vi "LIA Example Host.vi"() -> ()   [LabVIEW 2017]
uses:
  Program Files (x86)/National Instruments/LabVIEW 2017/examples/Lock-In Amplifier/lib/host/Public/pll settings.ctl
  Program Files (x86)/National Instruments/LabVIEW 2017/examples/Lock-In Amplifier/lib/host/Public/lock-in settings.ctl
  Program Files (x86)/National Instruments/LabVIEW 2017/examples/Lock-In Amplifier/lib/interface/Interface FPGA/LIA Host Interface FPGA.lvclass
  C:/Program Files (x86)/National Instruments/LabVIEW 2017/examples/Lock-In Amplifier/lib/interface/Interface/LIA Host Interface.lvclass
  Program Files (x86)/National Instruments/LabVIEW 2017/examples/Lock-In Amplifier/lib/host/Public/fpga type.ctl
  Program Files (x86)/National Instruments/LabVIEW 2017/examples/Lock-In Amplifier/lib/interface/Interface FPGA/Properties/FpgaSession_GET.vi
  <vilib>/Utility/error.llb/Error Cluster From Error Code.vi
  <vilib>/rvi/errors/niLvFpgaAdjustHostInterfaceError.vi
  <vilib>/rvi/interface/nirviReadWriteControl/nirviReadWriteControl.xnode
  Program Files (x86)/National Instruments/LabVIEW 2017/examples/Lock-In Amplifier/lib/interface/Interface/LIA Host Interface.lvclass
  Program Files (x86)/National Instruments/LabVIEW 2017/examples/Lock-In Amplifier/lib/host/Lock-In Amplifier Example Host.lvlib
  Program Files (x86)/National Instruments/LabVIEW 2017/examples/Lock-In Amplifier/lib/shared/Lock-In Amplifier Example Shared.lvlib
  NiFpgaLv.dll
  <vilib>/rvi/interface/Simulation/niFpgaSimulationCallBeginRW.vi
panel:
  in  "trigger slope 1":enum16{"Positive", "Negative"}(ring)
  in  "lowLevel 1":dbl caption="pll.q 2" format="%#_6f"
  in  "highLevel 1":dbl=0.25 caption="pll.q 2" format="%#_6f"
  in  "trigger slope 0":enum16{"Positive", "Negative"}(ring)
  in  "lowLevel 0":dbl caption="pll.q 2" format="%#_6f"
  in  "highLevel 0":dbl=0.25 caption="pll.q 2" format="%#_6f"
  out "pll.vco output 0":fxp<+/-,49,1>=0.5 format="%0^#1_8g"
  out "pll.q 2":dbl=0.5 format="%#_6pV"
  out "Waveform Graph":cluster{"f0":dbl, "df":dbl, "magnitude":dbl[]}[](graph)=[{"f0"=0.0, "df"=48828.125, "magnitude"=[-46.93833321413425, -48.890085398745086, -57.05864793570993, -63.948010145782, -57.10808944274945, -63.55723661730865, -57.477633254873524, -63.388970771981256, -57.83858653215573, -63.04278294236552, -58.310732731480286, -62.75659424633111, -59.01913953160205, -62.55034509450798, -59.76806715246457, -62.45290461669743, -60.67593939903783, -62.55360847730091, -61.80337052022501, -62.7503089432639, -62.95874542404657, -63.17666796807587, -64.24815178765463, -63.58179265883102, -65.96263589732504, -64.29834519828907, -67.76706631207706, -65.25530419899528, -69.69720964445415, -66.48978075872667, -72.0836829037614, -67.87758710008302, -74.95546090477261, -70.02468767091023, -78.46318325872932, -72.61789596314395, -82.74302220692796, -76.45363219872509, -86.93156331597662, -81.93411626073177, -89.39593580415576, -99.6170681323641, -88.66324403386615, -83.63767905833946, -86.78510178329685, -77.97514394138707, -83.83057336078254, -74.91042135055551, -81.5475507560879, -73.50059696206921, -78.86254697144325, -72.13420582514291, -77.68352683311363, -71.47125092202423, -75.95623700109, -71.27989762649543, -74.95441595981052, -71.25879209888319, -73.9595113284693, -71.56173669996721, -73.54477863881124, -72.29773534656574, -73.22367389861854, -72.96381308648769, -72.9988078797969, -73.86835428297962, -72.95305526553327, -75.2471462028992, -73.52456103236882, -76.90120154185578, -74.35415308379046, -78.75438807181995, -75.52159448517878, -81.97850502570516, -77.0522962144752, -83.72534671678167, -79.22667312669566, -87.72245228429632, -82.41997364153613, -92.98958808340201, -88.94092629488937, -99.50542487601304, -104.43928510750062, -96.68595945743522, -89.84335052432984, -91.19624554856414, -83.82262417189582, -90.01723416008254, -80.15754604679948, -85.81708298956508, -78.30065773404802, -85.06593198935606, -77.23628138343811, -82.71304646807387, -76.35856258445034, -81.61855339489769, -75.96594028137565, -80.15275231432624, -75.79741810419392, -78.97129025392613, -75.86427195094097, -78.17458456209165, -76.12085849656066, -77.85383262432903, -76.74912507995519, -77.25671541218556, -77.8982284228998, -77.8212535613011, -78.99364420828655, -77.9535986594113, -80.5765883437286, -78.71247862445587, -82.81330063919576, -79.90075393045993, -84.51582581828501, -80.84734822816016, -88.15097620058117, -83.06948686637503, -90.43795841683013, -87.05804894598725, -100.9044462888944, -91.16184483511006, -99.25318703849094, -113.00302254650566, -101.23938945826266, -94.74360211928621, -93.60935601063579, -86.60563663892235, -90.06499901122993, -82.85388280403822, -89.22123700503676, -81.17742163079215, -87.46988992571065, -80.0064748842741, -85.67242615027025, -79.5534829705813, -85.2386741467478, -78.36875630953557, -83.74067249570277, -78.58966459550572, -82.65136916700945, -78.45793002426842, -81.60291278830285, -78.78545275144468, -81.44873599291637, -79.46689782726857, -80.9546312968039, -80.34286350947234, -80.64680657897753, -81.40467594015718, -81.45416553874705, -82.91913176326895, -82.01356243362385, -84.4698494074905, -82.43677736126503, -86.83038860613686, -84.19971850756579, -89.09446672366998, -85.50637044704303, -93.27140345100959, -90.41560771649186, -102.15908510562295, -94.5879404286508, -103.56313351942903, -113.25509523061405, -96.25338657002342, -93.35849714429017, -94.3068008800362, -88.27873675614035, -93.30083233782412, -85.39601004639363, -91.46280056925573, -83.25477812069862, -89.43703075785405, -82.62438364466891, -88.2225308674539, -81.04566563419816, -87.59003295267959, -80.9135761936175, -85.77827427186253, -80.22308425470746, -85.54716936739837, -80.30173677397998, -84.2175901500595, -80.56732874040298, -83.37768242883448, -81.48306367425042, -83.8906905917171, -82.20138677185858, -83.36581337182099, -83.25360739403229, -83.86719108117094, -85.13623924398044, -84.60141920705034, -85.63247211425215, -84.61891754501954, -89.11219644534478, -86.93675308563888, -90.65086474060264, -86.91978227755536, -94.32232024107083, -91.1937031528676, -105.67835131078319, -96.01996999749672, -108.19743564556381, -102.1759528334099, -98.13408028328126, -95.42561864673883, -103.03927558417618, -93.13041820570994, -92.61599840933886, -87.41561823576637, -95.6167947640217, -85.45482114157137, -89.26172625327284, -83.64736821155725, -90.73728201983252, -82.95136175993244, -90.47704364999184, -83.00757026802304, -89.1024095672369, -82.29357706840872, -88.23475300940171, -82.03587331514377, -86.85968342180617, -82.35711341553477, -85.81709753106743, -82.79370712523529, -85.95880792378041, -84.08514911178878, -86.24056528669705, -84.26663563351609, -85.11149144200135, -85.48335371583636, -85.92142581813184, -86.91808359752399, -86.58865058087574, -89.98286982647136, -87.49532734785518, -91.95474837719652, -89.34803145467214, -94.49767349488376, -92.45873563416424, -108.8690430269248, -98.69933253742657, -105.06246392868492, -111.38768449697511, -96.99118510161742, -95.28935999072544, -99.57447315645048, -91.921208747929, -94.58067683198153, -89.26115689307557, -95.97632975434266, -87.71112562159823, -95.6026253040889, -86.8643653685995, -94.03413185014664, -84.75458821373303, -90.53152615195356, -84.18265238198386, -90.74003839355723, -83.81237200473785, -88.98630392767043, -83.46732671915824, -88.80833466935512, -84.3729693934194, -89.09540947774846, -84.11269221746572, -87.01477738659764, -85.46574647387061, -88.82633557926184, -85.30529533094341, -86.64432037411572, -88.38882956922036, -89.46178094867575, -88.65167305541695, -89.05173580146197, -90.56355933624823, -89.78350226994066, -93.12832102157176, -91.52067729309718, -99.30869554872353, -94.87507585179671, -103.34143765953752, -100.85184172648087, -122.81434116496578, -106.73815887001018, -100.4378952074342, -102.02001564406744, -97.52306851355098, -94.56940172267517, -96.76524495433301, -89.94805427338399, -97.3848170465787, -88.86035744990033, -94.19234755063327, -86.61835716903454, -91.20282103849767, -85.07595457318845, -91.55874293944323, -85.03788023396316, -91.60457024090475, -84.46215997256039, -90.57121250734171, -84.83435358765959, -90.33972168032196, -84.4873262300197, -89.24140029984238, -85.1352382372926, -88.70896083363503, -85.5975672934432, -89.12875853347873, -86.53505382308096, -89.60175411890748, -88.0071551620068, -89.28181547323886, -89.27126299467224, -89.37796771473032, -91.7125863209184, -91.52209806412742, -93.2645811544421, -91.18984143652762, -95.81363430158875, -93.62301569519619, -104.16775936541315, -104.90602312527591, -113.16700957432688, -116.28917731958283, -101.96572273705183, -98.41482687439297, -99.72098919139918, -94.22144853044513, -95.01564070694563, -94.17707694153272, -94.02287362186925, -89.58355059750363, -98.92261465033643, -89.02859420719695, -94.68073466314038, -86.44103147442705, -91.90373963098203, -86.4749062880022, -94.84153506645869, -86.32943545083764, -91.60215019601517, -86.2323824481995, -92.02155272951049, -85.9972623610034, -91.32387548251664, -85.588514296591, -91.53470648146998, -86.2096134918317, -90.35669055111491, -88.00287392840076, -90.12141751973901, -89.44766457872662, -91.62087976611487, -91.05208067549513, -92.06362797535392, -91.10989004012806, -92.02930632263177, -97.8326419437665, -100.36369914302273, -96.71323750153027, -96.77554535749293, -104.0483458530803, -100.02615902224633, -107.35748572388934, -107.18491846666, -111.2107942940795, -101.34493721885849, -96.18458817889217, -95.05818354852602, -97.34815447051216, -92.36349598065061, -95.78385348959006, -89.7086230203063, -93.2365210743273, -88.04737944359495, -95.39968104514571, -88.1751912031278, -94.33963358398256, -86.96835690829943, -94.3448391909962, -87.94543163312412, -92.90493597746648, -87.22030009538193, -92.61262896853015, -86.30586131244313, -91.96103440057696, -86.7710521640438, -92.10322890271088, -88.8099510544229, -93.31727026496762, -88.39915058817098, -92.9724660735097, -89.53892755878542, -93.5679390287161, -92.14368535308965, -93.89854406383924, -93.06540499762073, -95.3716098006777, -96.36846381712701, -93.63623239819597, -99.39911564797553, -98.40395825782761, -100.94269872968796, -100.48369232950719, -104.96898067375994, -114.335263021867, -101.40187975001979, -98.65627818089435, -106.58072970493392, -104.44376560744413, -95.83027356701794, -92.97753215916143, -101.26434292825368, -93.50367975283709, -93.37263244117777, -89.44861935863923, -95.343734550422, -89.99933130658839, -99.99527004643943, -88.94925644025324, -93.18301244517464, -88.50885338097075, -95.18084024984185, -87.20676030200416, -95.23926810467589, -87.09957224800853, -92.1757639701081, -88.10417272814877, -94.72106133839601, -87.7772108681502, -92.91109610741583, -89.72414668122461, -93.22742894203847, -91.63186037346222, -95.68890880122552, -90.18179583705027, -93.59223328781121, -92.50281370390375, -94.04741609159348, -95.5573835037378, -97.19098591462304, -99.76079766259453, -98.20546781981285, -120.67183723001071, -103.20327161610481, -117.22027024101293, -105.09645279442447, -111.76755429121258, -113.04120386427974, -100.65061200309104, -96.88654432109547, -94.60215846035042, -93.49825828753863, -97.1667542174504, -94.38236741729683, -96.783281591943, -92.939285616442, -95.42524341021134, -89.7310231461323, -96.61418552254929, -89.15181635406329, -93.97977001970317, -89.25630669378194, -99.16812248160959, -89.40549989469969, -97.02103373489075, -88.08117642000238, -96.17212999699518, -87.76166390724612, -93.64057438170258, -88.20421502757773, -94.63414445257587, -89.48275213078753, -92.03704873153879, -91.18822814375747, -94.02753580779823, -92.25046023804195, -94.18472031424919, -95.7912337432503, -97.17361952054567, -97.57189526176677, -96.93431865585318, -102.04551967744064, -98.01984334480733, -97.80936648544454, -96.58319851428925, -103.08073994551233, -110.00167882027728, -108.52196994994446, -105.04853402419212, -101.33233085003278, -100.05040433917165, -99.22073393358865, -97.90929268980324, -98.89113225851989, -94.89288879112064, -97.93384172752636, -93.22419277669928, -96.01960899562502, -90.96253017735826, -94.32065948649546, -90.18255956439114, -94.9243761616897, -88.73145096365911, -95.65826240076106, -90.10091760259287, -98.3156872459785, -88.97172432282879, -94.68357816611993, -89.22286435681411, -96.33113850492892, -90.27256468692858, -97.52356475116345, -92.28994918400562, -96.39548763580854, -90.89270553951194, -95.24683746449244, -92.28348737753878, -94.54135448918169, -92.42301671907596, -96.24508547590521, -99.44340135136264, -100.90085793594595, -101.8210082553093, -100.62139348876947, -107.75005082456524, -101.18792193308998, -100.62321402005587, -106.14445292006377, -105.83949578053429, -107.80632506741767, -102.54660223569036, -108.59151037419879, -96.90782677416453, -100.64769899514724, -98.90076837905437, -96.2725953153946, -100.63869480989204, -93.57497128631536, -97.48996544980523, -92.0598771078806, -97.43531529596639, -91.70896750245781, -97.62553199959177, -89.90453042801695, -98.1895558530371, -91.28563260418011, -96.58606769664732, -89.6602652167721, -97.63127451658008, -90.06188532337133, -96.88320254636814, -92.10434711550748, -102.83415328605342, -91.97522523546786, -96.69674529333655, -91.54555505247494, -96.45677376279522, -94.40105972915326, -99.06442453405175, -95.85784268220618, -100.11209838032768, -96.3666970525114, -100.25033668665256, -101.63701920876531, -101.33176509769909, -108.49220907293285, -105.20698869391131, -108.51201611499555, -110.56213658974848, -103.88286882354619, -107.29652775251672, -100.21199149373265, -102.84474849090422, -105.38837926677445, -101.63659463064025, -100.19927788160382, -95.8841790949619, -99.06159894948496, -93.83003777289345, -98.62241277299339, -93.41972484372512, -96.85163908187218, -92.22305012467251, -98.30931966050954, -91.01393465151821, -96.6610842279197, -93.01366348474153, -99.40254068724771, -91.98688250178945, -97.8197024210045, -90.34022028730962, -95.26212499971268, -90.48623787418245, -97.28501156955554, -93.02707841894987, -99.4242294058617, -93.78403579509337, -102.4058010943352, -92.81743718612427, -97.25554725609649, -97.04610938164143, -104.56111849036819, -101.9867276361093, -103.69614871490393, -104.74168040294428, -100.60066394657342, -102.48071416087461, -104.83064451058839, -107.26658041556234, -110.00503214084297, -103.90297408190925, -109.56149727793942, -103.52026679181287, -103.90051784161805, -102.01215965881818, -103.34803834159351, -98.0276145235799, -96.38035775134539, -97.3546077254475, -94.31453760099365, -99.30006326184404, -96.25250684947787, -96.12470450005495, -91.57830601960927, -94.56483812993685, -91.7611403679199, -100.05865004766831, -92.84402279338929, -95.8657101518119, -91.81837191684286, -96.8413097745885, -89.99396126510099, -100.6611154167793, -93.47882774662997, -101.6552886734432, -91.90487651880966, -97.29970250454008, -95.48622404677303, -100.41640918017757, -94.80515000968441, -98.5276945872201, -100.73609481029864, -98.04340547902302, -96.88540783402982, -103.44300868430581, -99.6601137575993, -104.35594220885358, -109.94922945338091, -109.10632479160674, -107.76641232941655, -105.2450226453189, -99.91265402083279, -99.95270124336952, -101.3299547913052, -99.96894232524801, -100.36365349460627, -102.86784602376038, -98.02737777122191, -96.17199616892495, -96.8931790371181, -95.96337763969792, -97.57196266275315, -95.0155693239098, -97.04855005360989, -94.47249259707691, -99.4517730137364, -92.94791202171595, -97.78312777875891, -94.30168526906485, -94.86398262799752, -93.54115309153002, -99.87583067187317, -92.51726891229963, -102.13604597983688, -92.17994531242135, -101.63856277413217, -95.35318079876619, -99.29709984960036, -95.35866979801156, -103.51166947626271, -94.86370220831154, -101.60407867882681, -103.74156718150365, -110.73370380070999, -103.71760139847281, -107.37490721838113, -109.9542240510403, -116.25403765775846, -108.23241740959084, -105.09846687198814, -105.44052253244195, -115.24118791748435, -103.49001515992114, -110.71286352533042, -105.89441442611357, -110.16493279526881, -99.82773652058825, -98.97179081977004, -98.45757481371732, -98.24962705928117, -96.73193799282699, -96.5175230963137, -96.15492740611579, -95.37412981355675, -103.58492432555138, -95.34117451236305, -97.11997617370957, -93.47520800696678, -110.25299719363927, -96.81885358127444, -99.9145312135518, -94.20482495341496, -98.89579295580432, -93.36303704542247, -100.68935843408086, -93.24714444319031, -100.69789100599222, -95.91175346020901, -104.76997205430096, -94.51143912041329, -100.54159089868858, -102.05805669840157, -99.78073889500477, -95.8994839656266, -104.44581361115654, -97.35459561709312, -102.43458217795424, -99.94756951585332, -116.63154202021275, -104.67083143207799, -105.9908001506922, -110.38171109041919, -112.65697869449573, -108.99847694028415, -108.57898585331196, -104.24393364688189, -105.73441833654073, -109.05313569411014, -109.36295935913135, -98.16710161937883, -100.71703118273305, -99.09017072666417, -99.65556811710037, -99.82196229518456, -96.7135911059506, -102.93949494534098, -98.73450476723507, -97.07204978552434, -94.0346238995044, -101.15510126297552, -96.31490423262902, -97.71794077324151, -95.06125394279763, -97.42135900154832, -93.74600546845856, -114.1734093772797, -94.81930930716295, -97.06186795913504, -97.8835566026099, -103.92592509446062, -93.22500956494437, -99.20608880696017, -96.85801972443574, -107.87319613965472, -95.4606711561285, -109.77479647459404, -101.94651160973874, -109.21384119060488, -103.26877357606884, -104.34360525896628, -103.21689879150107, -103.51193808052379, -110.73067516385558, -106.23572152985658, -100.40039512525607, -104.4691097545222, -101.492896976522, -108.0496930826297, -104.38836363424356, -103.20083256140792, -98.90311658646465, -112.5916141563029, -97.44686284058668, -98.65253112982872, -97.56094346469311, -99.80658861772346, -99.20048346610903, -96.35632860142131, -99.28522795713639, -98.60285966904206, -97.78263171380898, -95.6007337511918, -103.2099329489675, -95.38702929874557, -102.13771129182885, -95.14930315850044, -98.3128670125364, -92.63546383992049, -104.71027133304193, -96.912283335093, -108.90993472372125, -99.55733899189684, -105.52550816632844, -97.40882660368159, -104.42281900752256, -99.57292672864625, -100.7966736295322, -97.52156624066522, -99.99073018359479, -99.0509840665854, -101.68754399107273, -101.12194458233189, -102.0463932610904, -105.91609044634541, -113.23554586573385, -101.98602750398949, -105.2635176386883, -103.79769775471262, -105.9111241296442, -107.9342434738976, -100.92121390473184, -97.12092290766883, -102.37764998835347, -98.6487783972021, -106.87222299917964, -99.33800557071586, -101.79953571256968, -100.91730518889514, -98.78879349468048, -98.23175546624212, -97.00117266559471, -101.37082956877207, -96.83259964822547, -104.87830362769942, -98.16713025626292, -101.96039957310882, -96.50507041796234, -101.8071196906989, -95.79349732553376, -102.02735914214256, -97.56201616761655, -103.1907064807159, -100.09953975957055, -112.56599817646672, -96.53563750179535, -99.9094561567417, -104.40141402751925, -115.46650328556561, -99.71467979897997, -102.79169020107405, -115.69624536220817, -100.76234254160234, -101.71038578591319, -103.75525178434926, -109.55422465835552, -106.65763594732093, -100.05230601631467, -102.10477478530564, -107.51891686962597, -114.58223661159585, -103.67146489337358, -101.5653675539541, -102.32103991938665, -103.67558252237892, -105.48352665247177, -109.55108760057558, -100.02982943314349, -98.13628340653156, -99.47346703290722, -98.92228326973435, -106.95782992135295, -105.89070869451947, -100.44660814326556, -97.09766369078704, -107.64297990254909, -105.84369355013555, -99.08393974061082, -96.374032771269, -102.65269590892945, -97.64870380479474, -105.90868162170571, -96.9898469284162, -105.2441700741264, -106.53146741239493, -106.46615178101108, -99.37447573772154, -109.39976410894721, -104.62921354447154, -101.87865689170566, -101.32860591590756, -114.43680707235822, -106.46190634887617, -113.36934474874106, -112.67163951557576, -102.66437005552562, -101.59964732308622, -122.77511747329424, -105.70845427584239, -108.46107323638913, -122.08650568486307, -111.16233468390396, -105.6496162612092, -105.79716011047833, -109.29698973600742, -106.5972312190114, -106.38945639217272, -105.63454774600953, -110.2830820244838, -105.77280978659724, -108.93057545365407, -109.17523925675454, -104.7131107168997, -103.60696199900858, -102.73166871321888, -97.49220135377621, -99.78808799700637, -101.11339791104449, -105.3939613260955, -103.42765288248593, -105.9340205661671, -107.77841485489014, -112.54860851403683, -120.22611245470668, -103.24971407964512, -104.3429544521227, -107.19732309503469, -107.16251497679025, -108.44664442280767, -101.62190077250342, -111.55917555022586, -104.81037871139557, -102.19463977156316, -105.04595625851906, -111.13196253104579, -124.72753891569215, -106.41597417621414, -105.12116350513813, -109.07754889691405, -105.23915229069101, -100.2688134501812, -107.02689810915471, -109.80290323096122, -103.81257666065085, -103.93774311881742, -110.756399743658, -111.62163187481585, -104.70396973658701, -110.06008823269457, -102.37808137382835, -103.60682103116714, -108.7695179644936, -102.98806816979182, -108.95209477982092, -102.75152787003978, -110.5775345178838, -107.60670935161642, -111.40615158129323, -109.13401107224777, -116.61575163192845, -107.96409706790726, -107.25727436770623, -101.17937824997462, -101.48759426936303, -101.66993276693202, -108.51517738724363, -111.89027836420303, -105.82817808958634, -106.26049115128238, -115.0445929460676, -109.17008677215136, -110.56032445093282, -113.06962595211048, -104.72451144495747, -103.61986219276268, -103.93451254257806, -131.06358095275755, -105.10487085176783, -105.25246852224541, -106.12903690082682, -107.23522918531137, -106.27438688637619, -107.07518949090365, -106.0552389825976, -103.69306509532366, -103.41067687310449, -105.62796514613967, -105.09396645540701, -104.41575397097671, -106.21837017613421, -109.37322036445215, -107.2496046853047, -121.3348235662606, -111.11906633319107, -111.8877022511887, -112.63080142659376, -108.83825637747428, -106.2095359458504, -119.63268129656143, -123.9219371113987, -111.93522459359046, -111.31094152610274, -105.26691970177436, -106.04931130074439, -116.50378960248553, -113.82805948415167, -114.82071561851546, -107.43149967133049, -103.03687243275733, -101.63522623347686, -102.80934641992253, -107.82093212276692, -114.84037503828779, -112.35787341855624, -109.53816987092426, -102.9999489914469, -107.89601039792339, -106.37583865949857, -109.67283710223154]}, ...(4 in all)]
  in  "app.quit":bool
  in  "lock-in.boxcar length 0":u32=2048 caption="Boxar Length"
  in  "app.tab 0":enum32{"Lock-In", "PLL", "Output"}(tab)
  in  "lock-in.manual carrier 0":dbl=100000.0 caption="Carrier" format="%#_6p"
  in  "lock-in.decimation 0":i32=8192 caption="Decimation" min=8 max=8192
  in  "lock-in.source 0":enum16{"AI 0", "AI 1", "AI 2", "AI 3"}(ring)=enum."AI 1" caption="Channel"
  in  "lock-in.carrier 0":T1(ring)=enum."PLL 0" caption="Carrier Source"
  in  "pll.m 0":i8=-27 caption="M"
  in  "pll.source 0":enum16{"AI 0", "AI 1", "AI 2", "AI 3"}(ring) caption="Source"
  in  "pll.q frequency 0":dbl=100000.0 caption="Q Frequency" format="%#_6p"
  in  "pll.reset 0":bool
  in  "ao.noise 3":dbl caption="A0 3 Noise" min=0.0 max=1.0 format="%#_6p"
  in  "ao.level 3":dbl=0.5 caption="A0 3 Level" format="%#_6pV"
  in  "ao.frequency 3":dbl=10000000.0 caption="AO 3 Frequency" format="%#.9p"
  in  "ao.frequency 0":dbl=10000000.0 caption="AO 0 Frequency" format="%#.9p"
  in  "ao.level 0":dbl=0.5 caption="AO 0 Level" format="%#_6pV"
  in  "rio device":tag="PXI1Slot4" caption="Resource"
  in  "lock-in.reset boxar 0":bool
  out "lock-in.deviation 1":dbl caption="Deviation" format="%#_6p"
  out "lock-in.amplitude 0":dbl caption="Result" format="%#_6p"
  in  "lock-in.boxcar lookback 0":i32=1024 caption="Windows to Average"
  out "Result":cluster{"mean":dbl, "trace":dbl}(graph)
  # "pll.digital config 0"
  # "pll.digital config 1"
  # "NI Lock-In Amplifier Reference Example"
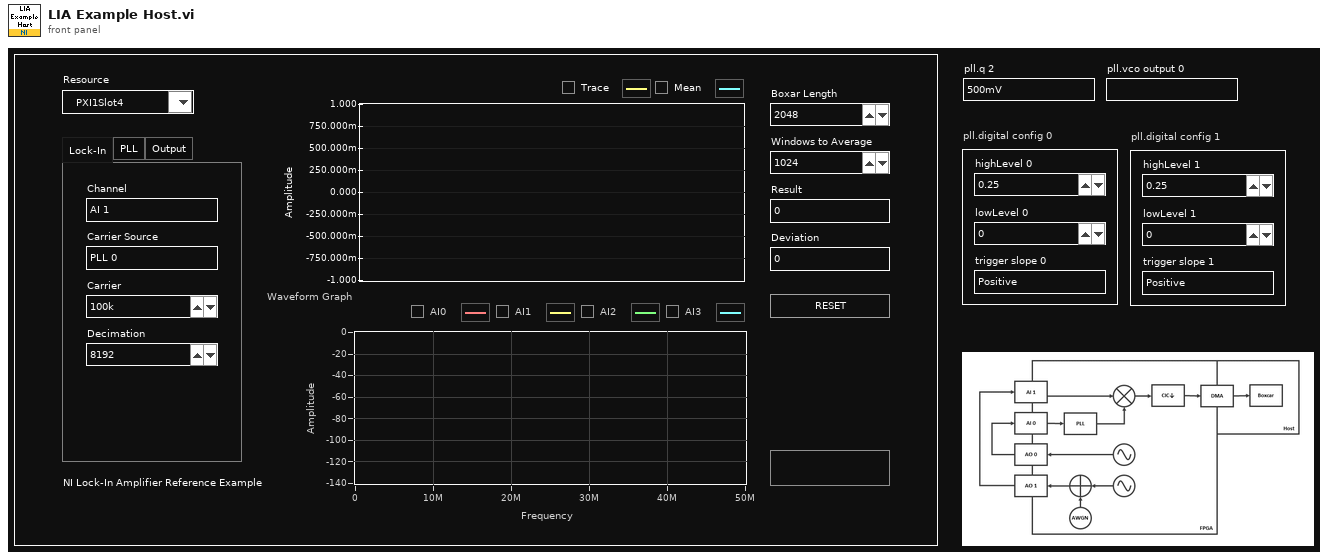
[diagram p1: front panel]
types:
  T1 = enum16{"Manual 0", "Manual 1", "Manual 2", "Manual 3", "PLL 0", "PLL 1"}
  T2 = typedef "Lock-In Amplifier Example Host.lvlib/lock-in settings.ctl" = cluster{"decimation":i32, "source":i32, "carrier source":i32, "carrier":dbl}
  T3 = typedef "Lock-In Amplifier Example Host.lvlib/pll settings.ctl" = cluster{"source":i32, "q frequency":dbl}
  T4 = cluster{"highLevel":fxp<+/-,18,1>, "lowLevel":fxp<+/-,18,1>, "trigger slope":enum8{"Positive", "Negative"}}
  T5 = typedef "Lock-In Amplifier Example Host.lvlib/fpga type.ctl" = refnum<k20>
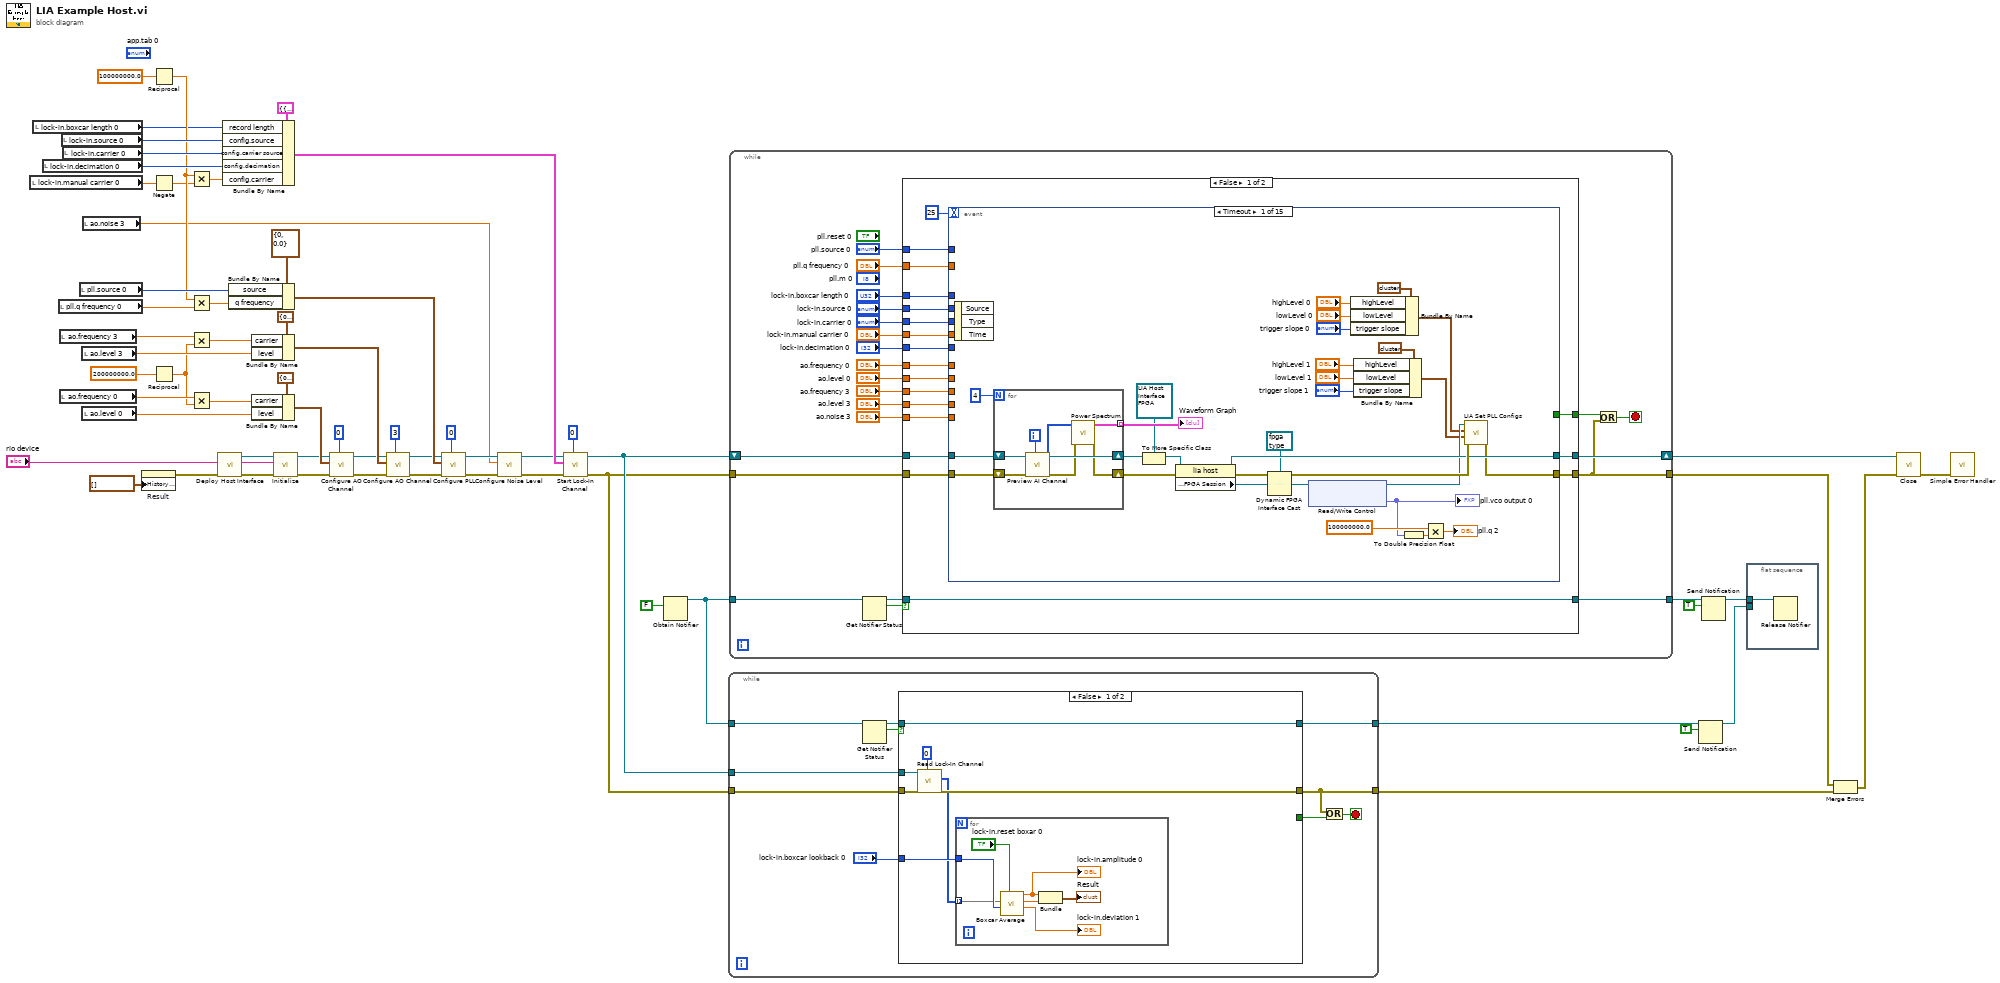
[diagram p0: block diagram]
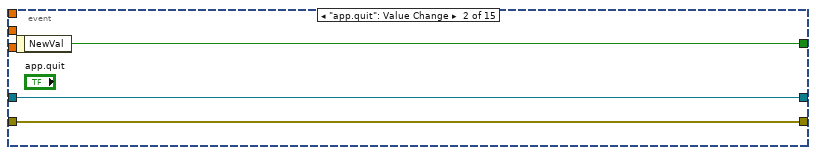
[diagram p2: hidden frame]
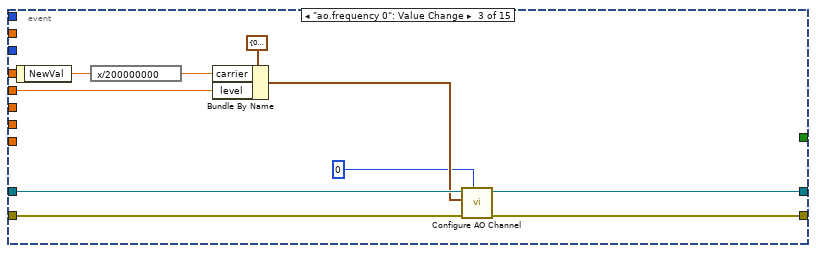
[diagram p3: hidden frame]
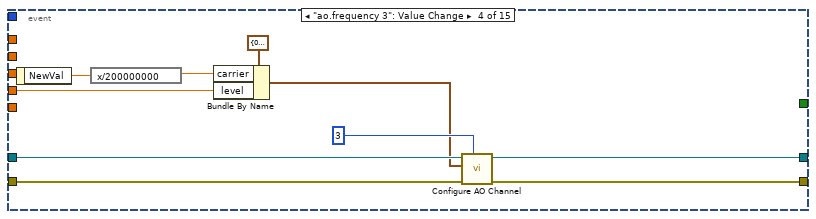
[diagram p4: hidden frame]
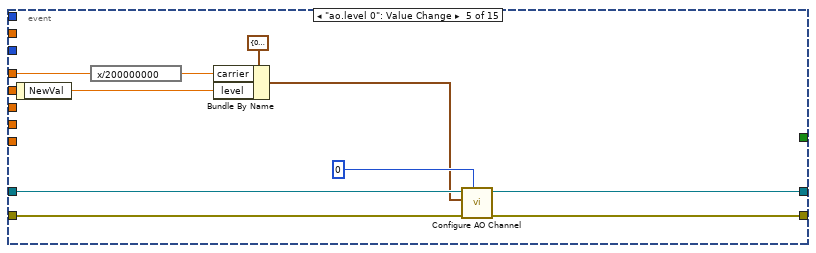
[diagram p5: hidden frame]
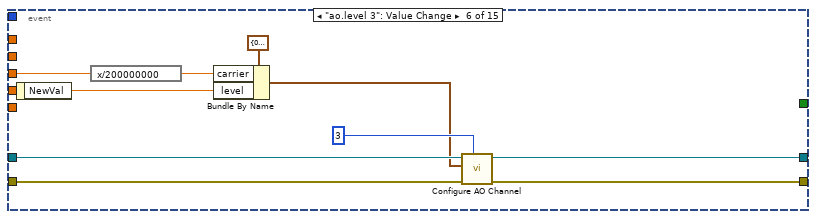
[diagram p6: hidden frame]
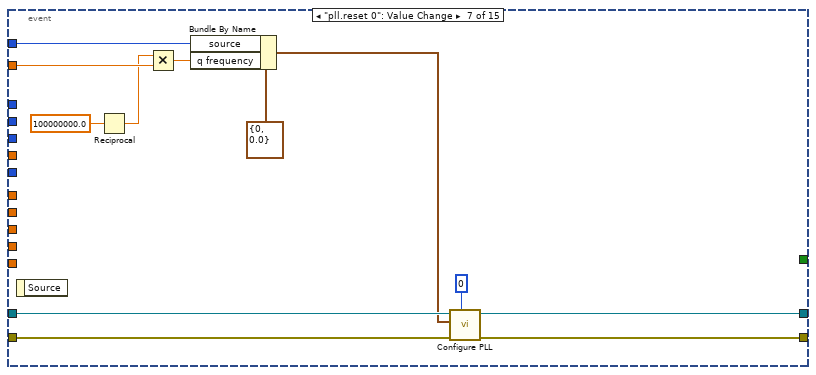
[diagram p7: hidden frame]
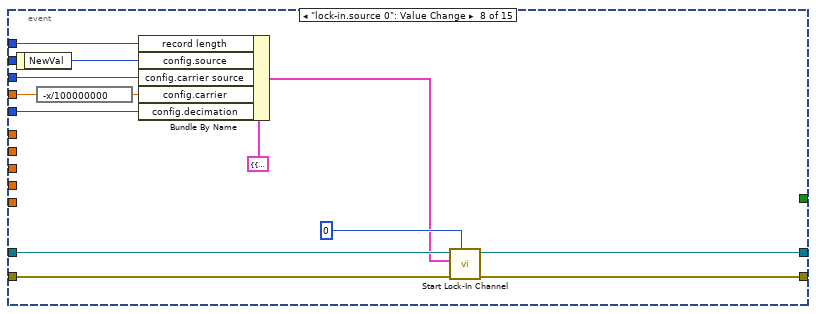
[diagram p8: hidden frame]
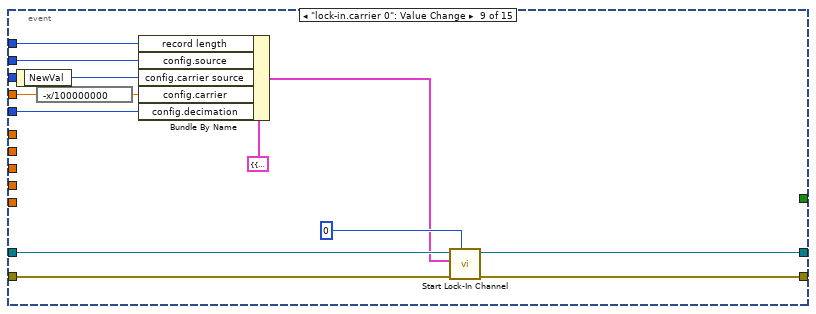
[diagram p9: hidden frame]
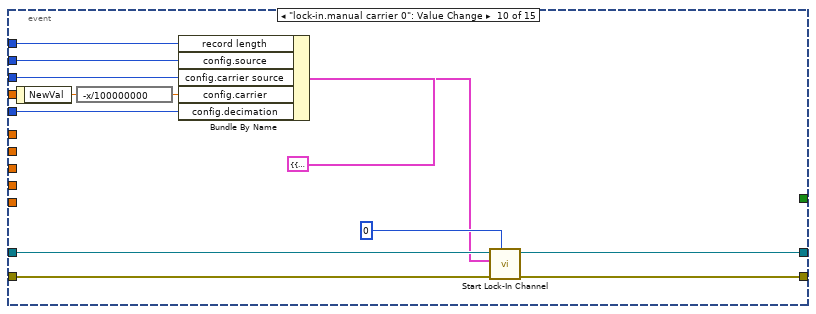
[diagram p10: hidden frame]
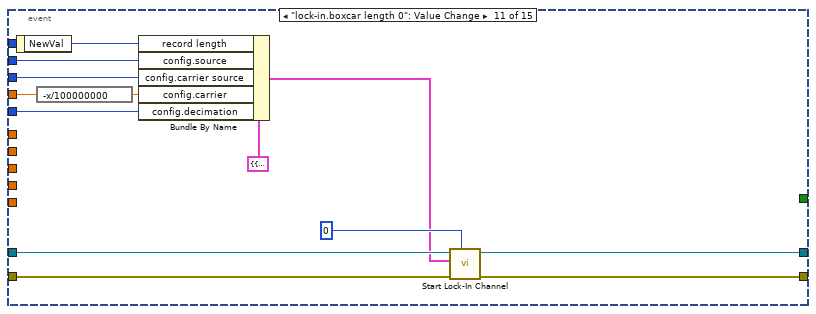
[diagram p11: hidden frame]
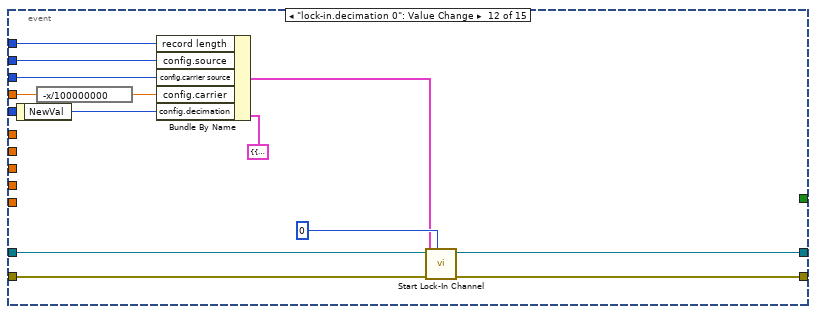
[diagram p12: hidden frame]
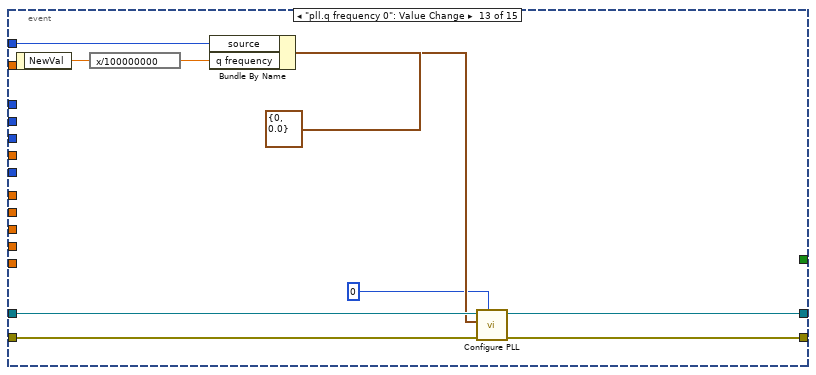
[diagram p13: hidden frame]
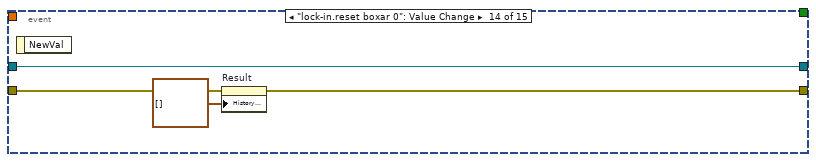
[diagram p14: hidden frame]
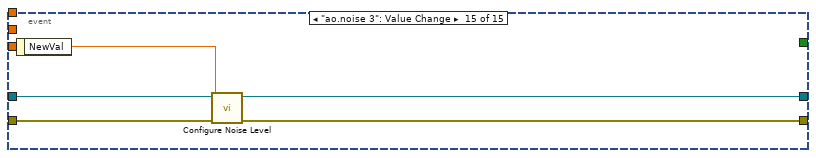
[diagram p15: hidden frame]
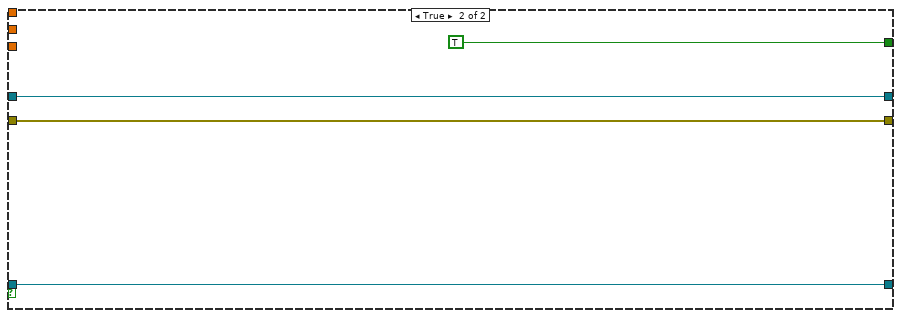
[diagram p16: hidden frame]
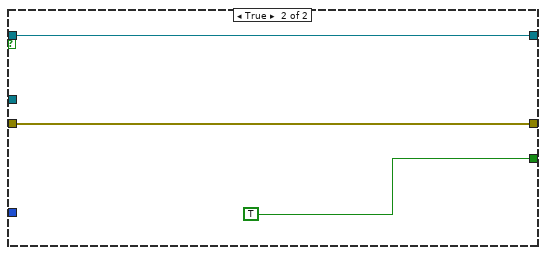
[diagram p17: hidden frame]
diagram:
  n1 = local read "lock-in.manual carrier 0"() -> (w50:dbl)
  n2 = local read "lock-in.boxcar length 0"() -> (w14:u32)
  n3 = local read "lock-in.decimation 0"() -> (w53:i32)
  n4 = local read "pll.q frequency 0"() -> (w55:dbl)
  n5 = local read "ao.frequency 3"() -> (w47:dbl)
  n6 = local read "ao.frequency 0"() -> (w44:dbl)
  n7 = local read "lock-in.source 0"() -> (w64:enum16{"AI 0", "AI 1", "AI 2", "AI 3"})
  n8 = local read "lock-in.carrier 0"() -> (w63:T1)
  n9 = local read "pll.source 0"() -> (w61:enum16{"AI 0", "AI 1", "AI 2", "AI 3"})
  n10 = local read "ao.level 3"() -> (w59:dbl)
  n11 = local read "ao.level 0"() -> (w58:dbl)
  n12 = local read "ao.noise 3"() -> (w3:dbl)
  n13 = property on="Result" class="WFChart (strict)"("History Data"=cluster{"mean":dbl, "trace":dbl}[] []) -> (error out=w9:errorcluster)  [unwired: 2 in, 1 out]
  n14 = Reciprocal(x=100000000.0) -> (1/x=w51:dbl)
  n15 = Negate(x=w50) -> (-x=w49:dbl)
  n16 = Reciprocal(x=200000000.0) -> (1/x=w43:dbl)
  n17 = Multiply(x=w51, y=w49) -> (x*y=w52:dbl)
  n18 = Multiply(x=w51, y=w55) -> (x*y=w56:dbl)
  n19 = Multiply(x=w47, y=w43) -> (x*y=w48:dbl)
  n20 = Multiply(x=w44, y=w43) -> (x*y=w45:dbl)
  n21 = call "Deploy Host Interface.vi"("error in"=w9, "resource"="rio device") -> ("error out"=w10:errorcluster, "resource out"=w11:string, "lia host interface"=w12:refnum<class "LIA Host Interface.lvclass">)  [unwired: 7 in]
  n22 = Bundle By Name(cluster=cluster{"config":T2, "record length":u32} {"config"={"decimation"=0, "source"=0, "carrier source"=0, "carrier"=0.0}, "record length"=0} ("config"), "record length"=w14, "config.source"=w64, "config.carrier source"=w63, "config.decimation"=w53, "config.carrier"=w52) -> (w15:cluster{"config":T2, "record length":u32})
  n23 = Bundle By Name(cluster=T3 {"source"=0, "q frequency"=0.0} ("config"), "source"=w61, "q frequency"=w56) -> (w40:T3)
  n24 = Bundle By Name(cluster=cluster{"carrier":dbl, "level":dbl} {"carrier"=0.0, "level"=0.0} ("config"), "carrier"=w48, "level"=w59) -> (w41:cluster{"carrier":dbl, "level":dbl})
  n25 = Bundle By Name(cluster=cluster{"carrier":dbl, "level":dbl} {"carrier"=0.0, "level"=0.0} ("config"), "carrier"=w45, "level"=w58) -> (w42:cluster{"carrier":dbl, "level":dbl})
  n26 = call-dynamic "Initialize.vi"("error in"=w10, "resource"=w11, "lia host in"=w12) -> ("error out"=w24:errorcluster, "lia host out"=w25:refnum<class "LIA Host Interface.lvclass">)  [unwired: 7 in]
  n27 = call-dynamic "Configure AO Channel.vi"("instance"=0 ("index"), "error in"=w24, "config"=w42, "lia host in"=w25) -> ("error out"=w23:errorcluster, "lia host out"=w22:refnum<class "LIA Host Interface.lvclass">)  [unwired: 6 in]
  n28 = call-dynamic "Configure AO Channel.vi"("instance"=3 ("index"), "error in"=w23, "config"=w41, "lia host in"=w22) -> ("error out"=w18:errorcluster, "lia host out"=w19:refnum<class "LIA Host Interface.lvclass">)  [unwired: 6 in]
  n29 = call-dynamic "Configure PLL.vi"("instance"=0 ("index"), "error in"=w18, "config"=w40, "lia host in"=w19) -> ("error out"=w7:errorcluster, "lia host out"=w4:refnum<class "LIA Host Interface.lvclass">)  [unwired: 6 in]
  n30 = call-dynamic "Configure Noise Level.vi"("error in"=w7, "level"=w3, "lia host in"=w4) -> ("error out"=w6:errorcluster, "lia host out"=w5:refnum<class "LIA Host Interface.lvclass">)  [unwired: 7 in]
  n31 = call-dynamic "Start Lock-In Channel.vi"("instance"=0 ("index"), "error in"=w6, "config"=w15, "lia host in"=w5) -> ("error out"=w35:errorcluster, "lia host out"=w36:refnum<class "LIA Host Interface.lvclass">)  [unwired: 6 in]
  n32 = Obtain Notifier(notification data type=FALSE) -> (notifier out=w37:refnum<notifier>)  [unwired: 3 in, 2 out]
  n33 = while {
    tunnel: w37 -> [w74]
    tunnel: w36 -> [w71]
    tunnel: w35 -> [w70]
    tunnel: [w69] -> w28
    tunnel: [w66] -> w31
    stop <- w68 stop-if-true
    n34 = Get Notifier Status(notifier=w74) -> (notifier out=w72:refnum<notifier>, current notification=w73:bool)  [unwired: 1 in, 3 out]
    n35 = case shown="False" w73 {
      tunnel: [w78 w91] -> w66
      tunnel: w72 -> [w78 w91]
      tunnel: w71 -> [w81 _]
      tunnel: w70 -> [w80 w90]
      tunnel: [w77 w90] -> w69
      tunnel: [_ TRUE] -> w67
      tunnel: "lock-in.boxcar lookback 0" -> [w76 _]
      frame False {
        n36 = call-dynamic "Read Lock-In Channel.vi"("instance"=0 ("index"), "error in"=w80, "lia host in"=w81) -> ("error out"=w77:errorcluster, "unscaled data"=w75:i64[][])  [unwired: 6 in, 1 out]
        n37 = for {
          tunnel: w75 -> [w83] mode=indexing
          tunnel: w76 -> [w84]
          n38 = call "Boxcar Average.vi"("reset"="lock-in.reset boxar 0", "sample length"=w84, "interleaved iq"=w83) -> ("standard deviation"=→"lock-in.deviation 1":dbl, "trace"=w88:dbl, "mean"=w85:dbl)  [unwired: 6 in]
          "lock-in.amplitude 0" <- w85
          n39 = Bundle("mean"=w85, "trace"=w88) -> (→"Result":cluster{"mean":dbl, "trace":dbl})  [unwired: 1 in]
        }
      }
      frame True {
      }
    }
    n40 = Or(x=w69, y=w67) -> (x .or. y?=w68:bool)
  }
  n41 = while {
    tunnel: w35 -> [w113]
    shift-right: [w99] -> w39
    shift-left: w36 -> [w112]
    tunnel: [w95] -> w27
    tunnel: w37 -> [w98]
    tunnel: [w93] -> w34
    stop <- w111 stop-if-true
    n42 = Get Notifier Status(notifier=w98) -> (notifier out=w97:refnum<notifier>, current notification=w96:bool)  [unwired: 1 in, 3 out]
    n43 = case shown="False" w96 {
      tunnel: w113 -> [w132 w311]
      tunnel: w112 -> [w131 w312]
      tunnel: [w130 w311] -> w95
      tunnel: "lock-in.manual carrier 0" -> [w128 _]
      tunnel: "lock-in.decimation 0" -> [w127 _]
      tunnel: "lock-in.source 0" -> [w126 _]
      tunnel: "lock-in.carrier 0" -> [w125 _]
      tunnel: "pll.source 0" -> [w124 _]
      tunnel: "pll.q frequency 0" -> [w123 _]
      tunnel: "ao.frequency 0" -> [w122 _]
      tunnel: "ao.level 0" -> [w121 _]
      tunnel: "ao.frequency 3" -> [w120 _]
      tunnel: "ao.level 3" -> [w119 _]
      tunnel: "ao.noise 3" -> [w118 _]
      tunnel: [w117 w312] -> w99
      tunnel: w97 -> [w115 w309]
      tunnel: [w116 TRUE] -> w94
      tunnel: [w115 w309] -> w93
      tunnel: "lock-in.boxcar length 0" -> [w114 _]
      frame False {
        n44 = event shown="[0] Timeout" {
          selector: _ -> [_ _ _ _ _ _ _ _ _ _ _ _ _ _ _]
          dyn-events: _ -> [_ _ _ _ _ _ _ _ _ _ _ _ _ _ _]
          timeout: 25 -> [_ _ _ _ _ _ _ _ _ _ _ _ _ _ _]
          tunnel: w132 -> [w159 w171 w177 w192 w202 w212 w224 w233 w247 w260 w272 w286 w295 w303 w307]
          tunnel: w131 -> [w160 w172 w178 w191 w201 w211 w223 w231 w245 w258 w270 w284 w294 w300 w308]
          tunnel: [w149 w171 w175 w190 w200 w210 w222 w232 w246 w259 w271 w285 w292 w302 w305] -> w130
          tunnel: w126 -> [_ _ _ _ _ _ _ _ w238 w251 w264 w280 _ _ _]
          tunnel: w125 -> [_ _ _ _ _ _ _ w236 _ w262 w275 w288 _ _ _]
          tunnel: w128 -> [_ _ _ _ _ _ _ w235 w249 _ w274 w287 _ _ _]
          tunnel: w127 -> [_ _ _ _ _ _ _ w234 w248 w261 w273 _ _ _ _]
          tunnel: w124 -> [_ _ _ _ _ _ w217 _ _ _ _ _ w297 _ _]
          tunnel: w123 -> [_ _ _ _ _ _ w218 _ _ _ _ _ _ _ _]
          tunnel: w122 -> [_ _ _ _ w195 _ _ _ _ _ _ _ _ _ _]
          tunnel: w121 -> [_ _ w180 _ _ _ _ _ _ _ _ _ _ _ _]
          tunnel: w120 -> [_ _ _ _ _ w205 _ _ _ _ _ _ _ _ _]
          tunnel: w119 -> [_ _ _ w185 _ _ _ _ _ _ _ _ _ _ _]
          tunnel: w118 -> [_ _ _ _ _ _ _ _ _ _ _ _ _ _ _]
          tunnel: [w154 w172 w173 w183 w193 w203 w213 w230 w244 w257 w269 w283 w293 w300 w306] -> w117
          tunnel: [_ w170 _ _ _ _ _ _ _ _ _ _ _ _ _] -> w116
          tunnel: w114 -> [_ _ _ _ _ _ _ w226 w241 w254 _ w278 _ _ _]
          event Timeout {
            n45 = event-data() -> ()  [unwired: 1 in, 3 out]
            n46 = for {
              N: 4 -> [_]
              shift-right: [w167] -> w155
              shift-left: w160 -> [w169]
              shift-right: [w164] -> w158
              shift-left: w159 -> [w168]
              tunnel: [w162] -> w156 mode=indexing
              i -> [w166]
              n47 = call-dynamic "Preview AI Channel.vi"("instance"=w166, "error in"=w168, "lia host in"=w169) -> ("error out"=w165:errorcluster, "samples"=w163:i16[], "lia host out"=w167:refnum<class "LIA Host Interface.lvclass">)  [unwired: 6 in]
              n48 = call "Power Spectrum.vi"("error in"=w165, "ai data"=w163) -> ("error out"=w164:errorcluster, "magnitude"=w162:cluster{"f0":dbl, "df":dbl, "magnitude":dbl[]})  [unwired: 8 in]
            }
            "Waveform Graph" <- w156
            n49 = To More Specific Class(target class=refnum<class "LIA Host Interface FPGA.lvclass"> refnum ("lia host"), reference=w155) -> (specific class reference=w153:refnum<class "LIA Host Interface FPGA.lvclass">)  [unwired: 1 in, 1 out]
            n50 = property class="lia host"(reference=w153, error in=w158) -> (reference out=w154:refnum<class "LIA Host Interface FPGA.lvclass">, error out=w161:errorcluster, "Properties:FPGA Session"=w151:refnum<k20>)
            n51 = Dynamic FPGA Interface Cast(Session In=T5 refnum ("fpga type"), Type=w151) -> (Session Out=w148:T5)
            n52 = xnode "Read/Write Control"("FPGA VI Reference In"=w148) -> ("FPGA VI Reference Out"=w144:T5, "pll.vco output 0"=w143:fxp<+/-,49,1>)  [unwired: 1 in, 1 out]
            "pll.vco output 0" <- w143
            n53 = Bundle By Name(cluster=T4 {"highLevel"=0.0, "lowLevel"=0.0, "trigger slope"=enum."Positive"} ("pll.digital config 0"), "highLevel"="highLevel 0", "lowLevel"="lowLevel 0", "trigger slope"="trigger slope 0") -> (w134:T4)
            n54 = Bundle By Name(cluster=T4 {"highLevel"=0.0, "lowLevel"=0.0, "trigger slope"=enum."Positive"} ("pll.digital config 0"), "highLevel"="highLevel 1", "lowLevel"="lowLevel 1", "trigger slope"="trigger slope 1") -> (w133:T4)
            n55 = To Double Precision Float(number=w143) -> (double precision float=w147:dbl)
            n56 = Multiply(x=100000000.0, y=w147) -> (x*y=→"pll.q 2":dbl)
            n57 = call "LIA Set PLL Configs.vi"("error in (no error)"=w161, "pll.digital config 1"=w133, "pll.digital config 0"=w134, "fpga session in"=w144) -> ("error out"=w149:errorcluster)  [unwired: 7 in]
          }
          event "app.quit": Value Change {
            n58 = event-data() -> ("NewVal"=w170:bool)  [unwired: 1 in]
          }
          event "ao.frequency 0": Value Change {
            n59 = event-data() -> ("NewVal"=w179:dbl)  [unwired: 1 in]
            n60 = expression code="x/200000000"(w179) -> (w181:dbl)
            n61 = Bundle By Name(cluster=cluster{"carrier":dbl, "level":dbl} {"carrier"=0.0, "level"=0.0} ("config"), "carrier"=w181, "level"=w180) -> (w176:cluster{"carrier":dbl, "level":dbl})
            n62 = call-dynamic "Configure AO Channel.vi"("instance"=0 ("index"), "error in"=w177, "config"=w176, "lia host in"=w178) -> ("error out"=w175:errorcluster, "lia host out"=w173:refnum<class "LIA Host Interface.lvclass">)  [unwired: 6 in]
          }
          event "ao.frequency 3": Value Change {
            n63 = event-data() -> ("NewVal"=w186:dbl)  [unwired: 1 in]
            n64 = expression code="x/200000000"(w186) -> (w188:dbl)
            n65 = Bundle By Name(cluster=cluster{"carrier":dbl, "level":dbl} {"carrier"=0.0, "level"=0.0} ("config"), "carrier"=w188, "level"=w185) -> (w184:cluster{"carrier":dbl, "level":dbl})
            n66 = call-dynamic "Configure AO Channel.vi"("instance"=3 ("index"), "error in"=w192, "config"=w184, "lia host in"=w191) -> ("error out"=w190:errorcluster, "lia host out"=w183:refnum<class "LIA Host Interface.lvclass">)  [unwired: 6 in]
          }
          event "ao.level 0": Value Change {
            n67 = event-data() -> ("NewVal"=w196:dbl)  [unwired: 1 in]
            n68 = expression code="x/200000000"(w195) -> (w198:dbl)
            n69 = Bundle By Name(cluster=cluster{"carrier":dbl, "level":dbl} {"carrier"=0.0, "level"=0.0} ("config"), "carrier"=w198, "level"=w196) -> (w194:cluster{"carrier":dbl, "level":dbl})
            n70 = call-dynamic "Configure AO Channel.vi"("instance"=0 ("index"), "error in"=w202, "config"=w194, "lia host in"=w201) -> ("error out"=w200:errorcluster, "lia host out"=w193:refnum<class "LIA Host Interface.lvclass">)  [unwired: 6 in]
          }
          event "ao.level 3": Value Change {
            n71 = event-data() -> ("NewVal"=w206:dbl)  [unwired: 1 in]
            n72 = expression code="x/200000000"(w205) -> (w208:dbl)
            n73 = Bundle By Name(cluster=cluster{"carrier":dbl, "level":dbl} {"carrier"=0.0, "level"=0.0} ("config"), "carrier"=w208, "level"=w206) -> (w204:cluster{"carrier":dbl, "level":dbl})
            n74 = call-dynamic "Configure AO Channel.vi"("instance"=3 ("index"), "error in"=w212, "config"=w204, "lia host in"=w211) -> ("error out"=w210:errorcluster, "lia host out"=w203:refnum<class "LIA Host Interface.lvclass">)  [unwired: 6 in]
          }
          event "pll.reset 0": Value Change {
            n75 = event-data() -> ()  [unwired: 1 in, 1 out]
            n76 = Reciprocal(x=100000000.0) -> (1/x=w215:dbl)
            n77 = Multiply(x=w215, y=w218) -> (x*y=w220:dbl)
            n78 = Bundle By Name(cluster=T3 {"source"=0, "q frequency"=0.0} ("config"), "source"=w217, "q frequency"=w220) -> (w214:T3)
            n79 = call-dynamic "Configure PLL.vi"("instance"=0 ("index"), "error in"=w224, "config"=w214, "lia host in"=w223) -> ("error out"=w222:errorcluster, "lia host out"=w213:refnum<class "LIA Host Interface.lvclass">)  [unwired: 6 in]
          }
          event "lock-in.source 0": Value Change {
            n80 = event-data() -> ("NewVal"=w228:enum16{"AI 0", "AI 1", "AI 2", "AI 3"})  [unwired: 1 in]
            n81 = expression code="-x/100000000"(w235) -> (w237:dbl)
            n82 = Bundle By Name(cluster=cluster{"config":T2, "record length":u32} {"config"={"decimation"=0, "source"=0, "carrier source"=0, "carrier"=0.0}, "record length"=0} ("config"), "record length"=w226, "config.source"=w228, "config.carrier source"=w236, "config.carrier"=w237, "config.decimation"=w234) -> (w225:cluster{"config":T2, "record length":u32})
            n83 = call-dynamic "Start Lock-In Channel.vi"("instance"=0 ("index"), "error in"=w233, "config"=w225, "lia host in"=w231) -> ("error out"=w232:errorcluster, "lia host out"=w230:refnum<class "LIA Host Interface.lvclass">)  [unwired: 6 in]
          }
          event "lock-in.carrier 0": Value Change {
            n84 = event-data() -> ("NewVal"=w239:T1)  [unwired: 1 in]
            n85 = expression code="-x/100000000"(w249) -> (w250:dbl)
            n86 = Bundle By Name(cluster=cluster{"config":T2, "record length":u32} {"config"={"decimation"=0, "source"=0, "carrier source"=0, "carrier"=0.0}, "record length"=0} ("config"), "record length"=w241, "config.source"=w238, "config.carrier source"=w239, "config.carrier"=w250, "config.decimation"=w248) -> (w240:cluster{"config":T2, "record length":u32})
            n87 = call-dynamic "Start Lock-In Channel.vi"("instance"=0 ("index"), "error in"=w247, "config"=w240, "lia host in"=w245) -> ("error out"=w246:errorcluster, "lia host out"=w244:refnum<class "LIA Host Interface.lvclass">)  [unwired: 6 in]
          }
          event "lock-in.manual carrier 0": Value Change {
            n88 = event-data() -> ("NewVal"=w252:dbl)  [unwired: 1 in]
            n89 = expression code="-x/100000000"(w252) -> (w263:dbl)
            n90 = Bundle By Name(cluster=cluster{"config":T2, "record length":u32} {"config"={"decimation"=0, "source"=0, "carrier source"=0, "carrier"=0.0}, "record length"=0} ("config"), "record length"=w254, "config.source"=w251, "config.carrier source"=w262, "config.carrier"=w263, "config.decimation"=w261) -> (w253:cluster{"config":T2, "record length":u32})
            n91 = call-dynamic "Start Lock-In Channel.vi"("instance"=0 ("index"), "error in"=w260, "config"=w253, "lia host in"=w258) -> ("error out"=w259:errorcluster, "lia host out"=w257:refnum<class "LIA Host Interface.lvclass">)  [unwired: 6 in]
          }
          event "lock-in.boxcar length 0": Value Change {
            n92 = event-data() -> ("NewVal"=w265:u32)  [unwired: 1 in]
            n93 = expression code="-x/100000000"(w274) -> (w276:dbl)
            n94 = Bundle By Name(cluster=cluster{"config":T2, "record length":u32} {"config"={"decimation"=0, "source"=0, "carrier source"=0, "carrier"=0.0}, "record length"=0} ("config"), "record length"=w265, "config.source"=w264, "config.carrier source"=w275, "config.carrier"=w276, "config.decimation"=w273) -> (w266:cluster{"config":T2, "record length":u32})
            n95 = call-dynamic "Start Lock-In Channel.vi"("instance"=0 ("index"), "error in"=w272, "config"=w266, "lia host in"=w270) -> ("error out"=w271:errorcluster, "lia host out"=w269:refnum<class "LIA Host Interface.lvclass">)  [unwired: 6 in]
          }
          event "lock-in.decimation 0": Value Change {
            n96 = event-data() -> ("NewVal"=w281:i32)  [unwired: 1 in]
            n97 = expression code="-x/100000000"(w287) -> (w289:dbl)
            n98 = Bundle By Name(cluster=cluster{"config":T2, "record length":u32} {"config"={"decimation"=0, "source"=0, "carrier source"=0, "carrier"=0.0}, "record length"=0} ("config"), "record length"=w278, "config.source"=w280, "config.carrier source"=w288, "config.carrier"=w289, "config.decimation"=w281) -> (w277:cluster{"config":T2, "record length":u32})
            n99 = call-dynamic "Start Lock-In Channel.vi"("instance"=0 ("index"), "error in"=w286, "config"=w277, "lia host in"=w284) -> ("error out"=w285:errorcluster, "lia host out"=w283:refnum<class "LIA Host Interface.lvclass">)  [unwired: 6 in]
          }
          event "pll.q frequency 0": Value Change {
            n100 = event-data() -> ("NewVal"=w296:dbl)  [unwired: 1 in]
            n101 = expression code="x/100000000"(w296) -> (w299:dbl)
            n102 = Bundle By Name(cluster=T3 {"source"=0, "q frequency"=0.0} ("config"), "source"=w297, "q frequency"=w299) -> (w291:T3)
            n103 = call-dynamic "Configure PLL.vi"("instance"=0, "error in"=w295, "config"=w291, "lia host in"=w294) -> ("error out"=w292:errorcluster, "lia host out"=w293:refnum<class "LIA Host Interface.lvclass">)  [unwired: 6 in]
          }
          event "lock-in.reset boxar 0": Value Change {
            n104 = event-data() -> ()  [unwired: 1 in, 1 out]
            n105 = property on="Result" class="WFChart (strict)"(error in=w303, "History Data"=cluster{"mean":dbl, "trace":dbl}[] []) -> (error out=w302:errorcluster)  [unwired: 1 in, 1 out]
          }
          event "ao.noise 3": Value Change {
            n106 = event-data() -> ("NewVal"=w304:dbl)  [unwired: 1 in]
            n107 = call-dynamic "Configure Noise Level.vi"("error in"=w307, "level"=w304, "lia host in"=w308) -> ("error out"=w305:errorcluster, "lia host out"=w306:refnum<class "LIA Host Interface.lvclass">)  [unwired: 7 in]
          }
        }
      }
      frame True {
      }
    }
    n108 = Or(x=w94, y=w95) -> (x .or. y?=w111:bool)
  }
  n109 = Send Notification(notification=TRUE, notifier=w31) -> (notifier out=w29:refnum<notifier>)  [unwired: 1 in, 1 out]
  n110 = Send Notification(notification=TRUE, notifier=w34) -> (notifier out=w30:refnum<notifier>)  [unwired: 1 in, 1 out]
  n111 = flat-sequence {
    tunnel: w30 -> [w313]
    tunnel: w29 -> [_]
    frame #0 {
      n112 = Release Notifier(notifier=w313) -> ()  [unwired: 2 in, 3 out]
    }
  }
  n113 = Merge Errors(w27, w28) -> (w26:errorcluster)
  n114 = call-dynamic "Close.vi"("error in"=w26, "lia host in"=w39) -> ("error out"=w2:errorcluster)  [unwired: 8 in, 1 out]
  n115 = call <vilib>:"Simple Error Handler.vi"("error in (no error)"=w2) -> ()  [unwired: 4 in, 5 out]
